vi "length_checksum.vi"(1 "Input Byte Array":u8[](array[numeric])) -> (0 "Size byte + checksum":u8[](array[numeric]))   [LabVIEW 2012]
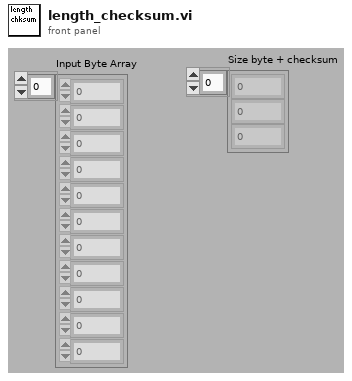
[diagram p1: front panel]
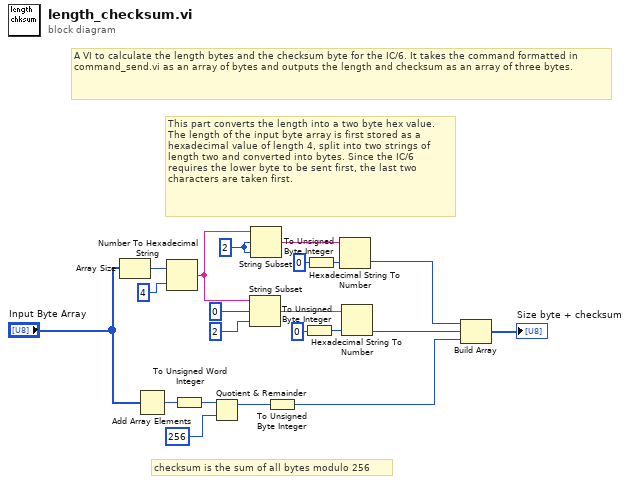
[diagram p0: block diagram]
diagram:
  w2 = 2
  # "This part converts the length into a two byte hex value. The length of the input byte array is first stored as a hexadecimal value of length 4, split into two strings of length two and converted into bytes. Since the IC/6 requires the lower byte to be sent first, the last two characters are taken first."
  # "checksum is the sum of all bytes modulo 256"
  # "A VI to calculate the length bytes and the checksum byte for the IC/6. It takes the command formatted in command_send.vi as an array of bytes and outputs the length and checksum as an array of three bytes."
  n1 = Array Size(array="Input Byte Array") -> (size(s)=w16:i32)
  n2 = Add Array Elements(numeric array="Input Byte Array") -> (sum=w20:u8)
  n3 = Number To Hexadecimal String(1:4, 2:w16) -> (0:w13:string)
  n4 = To Unsigned Word Integer(number=w20) -> (unsigned 16bit integer=w1:u16)
  n5 = Quotient & Remainder(x=w1, y=u16 256) -> (x-y*floor(x/y)=w18:u16)  [unwired: 1 out]
  n6 = String Subset(string=w13, offset (0)=0, length (rest)=2) -> (substring=w5:string)
  n7 = String Subset(string=w13, offset (0)=w2, length (rest)=w2) -> (substring=w12:string)
  n8 = To Unsigned Byte Integer(number=w18) -> (unsigned 8bit integer=w17:u8)
  n9 = To Unsigned Byte Integer(number=0) -> (unsigned 8bit integer=w7:u8)
  n10 = To Unsigned Byte Integer(number=0) -> (unsigned 8bit integer=w11:u8)
  n11 = Hexadecimal String To Number(string=w12, default (0uL)=w11) -> (number=w9:u8)  [unwired: 1 in, 1 out]
  n12 = Hexadecimal String To Number(string=w5, default (0uL)=w7) -> (number=w8:u8)  [unwired: 1 in, 1 out]
  n13 = Build Array(w9, w8, w17) -> (→"Size byte + checksum":u8[])
